vi "Calculate Team Ranking Positions.vi"(11 "Ranked Teams in":T1(array[cluster])) -> (2 "Rankings":string[](array[string]), 3 "Ranked Teams out":T1(array[cluster]))   [LabVIEW 2013]
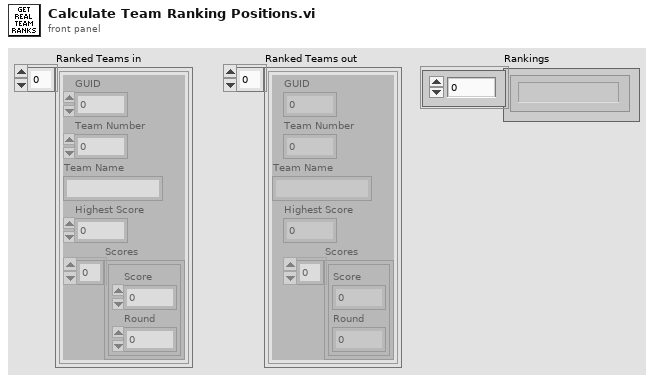
[diagram p1: front panel]
types:
  T1 = cluster{"GUID":u16, "Team Number":u16, "Team Name":string, "Highest Score":dbl, "Scores":cluster{"Score":dbl, "Round":u16}[]}[]
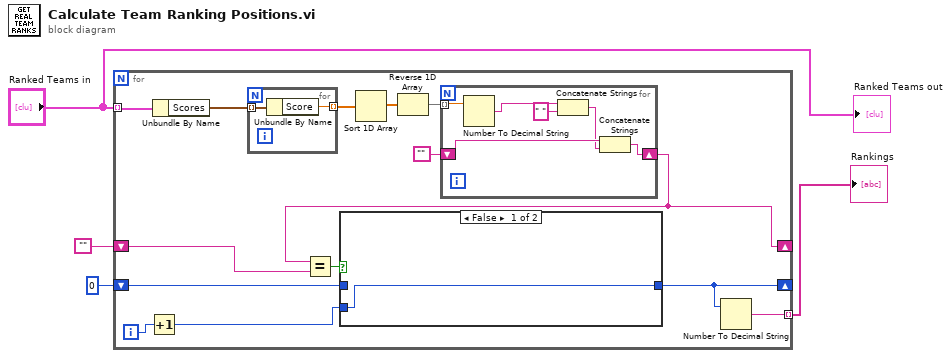
[diagram p0: block diagram]
diagram:
  n1 = for {
    tunnel: "Ranked Teams in" -> [w18] mode=indexing
    shift-right: [w7] -> _
    shift-left: "" -> [w8]
    shift-right: [w6] -> _
    shift-left: 0 -> [w10]
    tunnel: [w5] -> w2 mode=indexing
    i -> [w12]
    n2 = Increment(x=w12) -> (x+1=w11:i32)
    n3 = Unbundle By Name(w18) -> ("Scores"=w17:cluster{"Score":dbl, "Round":u16}[])
    n4 = for {
      tunnel: w17 -> [w28] mode=indexing
      tunnel: [w27] -> w16 mode=indexing
      n5 = Unbundle By Name(w28) -> ("Score"=w27:dbl)
    }
    n6 = Sort 1D Array(array=w16) -> (sorted array=w15:dbl[])
    n7 = Reverse 1D Array(array=w15) -> (reversed array=w14:dbl[])
    n8 = for {
      tunnel: w14 -> [w26] mode=indexing
      shift-right: [w21] -> w7
      shift-left: "" -> [w23]
      n9 = Number To Decimal String(number=w26) -> (decimal integer string=w25:string)  [unwired: 1 in]
      n10 = Concatenate Strings(w25, " " ("string")) -> (w22:string)
      n11 = Concatenate Strings(w23, w22) -> (w21:string)
    }
    n12 = Equal?(x=w7, y=w8) -> (x = y?=w9:bool)
    n13 = case shown="False" w9 {
      tunnel: w11 -> [w19 _]
      tunnel: w10 -> [_ w20]
      tunnel: [w19 w20] -> w6
      frame False {
      }
      frame True {
      }
    }
    n14 = Number To Decimal String(number=w6) -> (decimal integer string=w5:string)  [unwired: 1 in]
  }
  "Rankings" <- w2
  "Ranked Teams out" <- "Ranked Teams in"
